vi "Main.vi"(8 "error in (no error)":errorcluster, 10 "Temperature_Notifier":refnum<notifier>, 11 "Message Queues":T1) -> (0 "error out":errorcluster)   [LabVIEW 2019, in "USB-87P8_Manager.lvlib"]
uses:
  USB-87P8_Manager.lvlib
  Framework/Message Queue/All Message Queues.ctl
  Framework/Message Queue/Message Cluster.ctl
  Actor/USB-87Pn_Data.ctl
  USB-87Pn.lvclass
  <vilib>/Utility/sysdir.llb/System Directory Type.ctl
  Framework/Message Queue/Enqueue Message (Single).vi
  Framework/Message Queue/Message Queue.lvlib
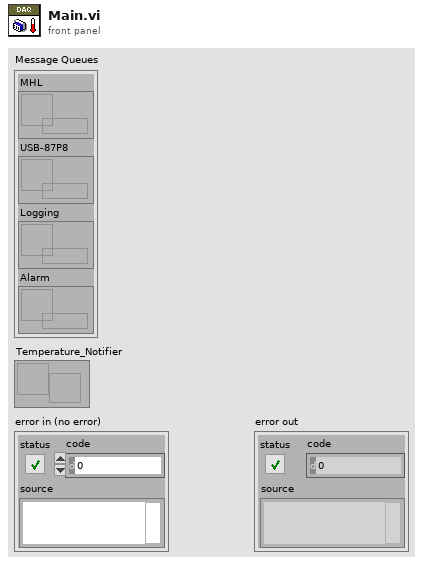
[diagram p1: front panel]
types:
  T1 = typedef "Message Queue.lvlib/All Message Queues.ctl" = cluster{"MHL":refnum<queue>, "USB-87P8":refnum<queue>, "Logging":refnum<queue>, "Alarm":refnum<queue>}
  T2 = typedef "USB-87P8_Manager.lvlib/USB-87Pn_Data.ctl" = cluster{"USB-87Pn":refnum<class "USB-87Pn.lvclass">, "Config_Base_Path":path, "COM Port":i32, "Running?":bool}
  T3 = typedef "System Directory Type.ctl" = i32
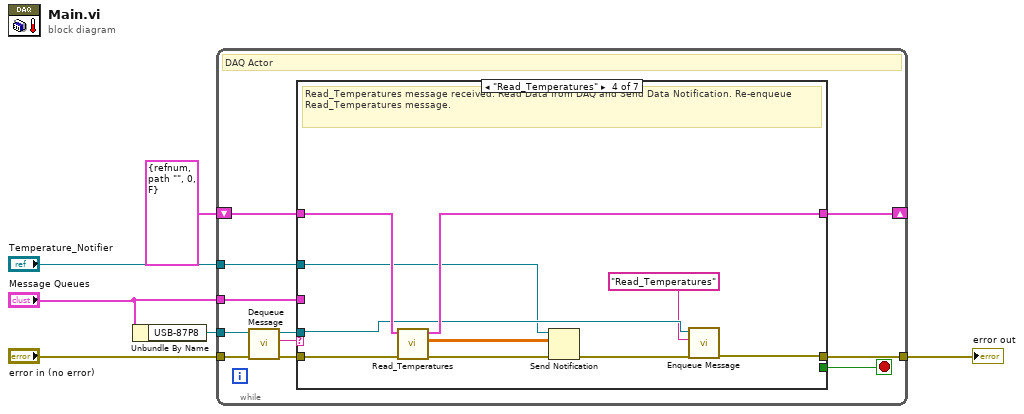
[diagram p0: block diagram]
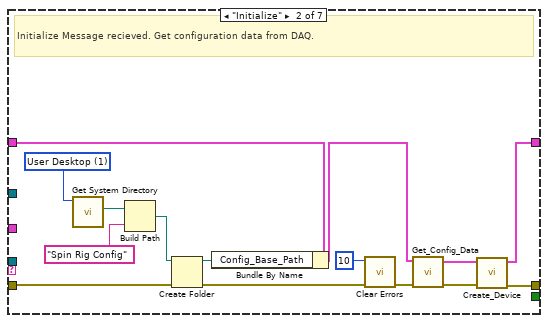
[diagram p3: hidden frame]
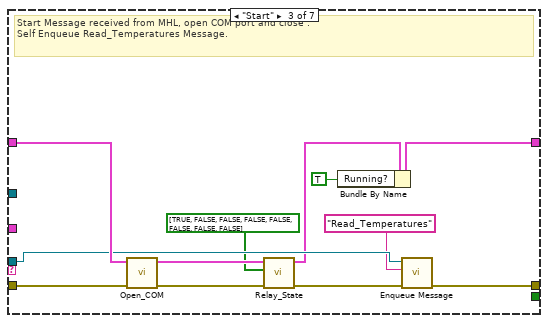
[diagram p4: hidden frame]
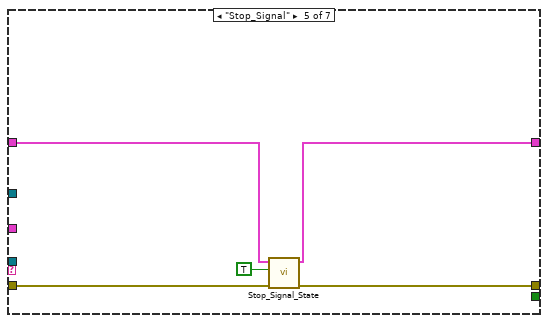
[diagram p5: hidden frame]
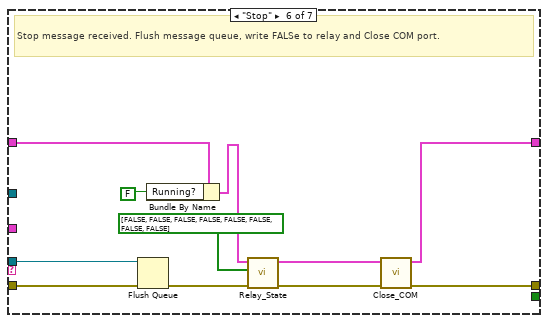
[diagram p6: hidden frame]
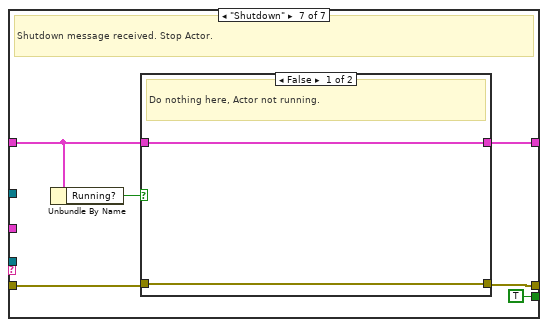
[diagram p7: hidden frame]
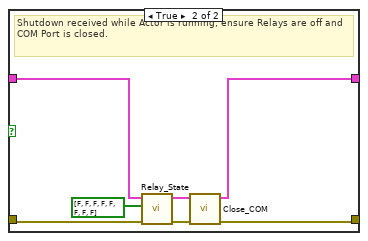
[diagram p8: hidden frame]
diagram:
  n1 = Unbundle By Name("Message Queues") -> ("USB-87P8"=w4:refnum<queue>)
  n2 = while {
    tunnel: "error in (no error)" -> [w17]
    tunnel: "Message Queues" -> [w12]
    tunnel: w4 -> [w16]
    tunnel: [w11] -> w3
    shift-right: [w8] -> _
    shift-left: T2 {"USB-87Pn"=refnum, "Config_Base_Path"=path "", "COM Port"=0, "Running?"=FALSE} -> [w9]
    tunnel: "Temperature_Notifier" -> [w7]
    stop <- w10 stop-if-true
    # "DAQ Actor"
    n3 = call "Dequeue Message.vi"("error in (no error)"=w17, "Message Queue"=w16) -> ("error out"=w13:errorcluster, "Message"=w14:string, "dup Message Queue"=w15:refnum<queue>)  [unwired: 6 in, 1 out]
    n4 = case shown="\"Read_Temperatures\"" w14 {
      tunnel: w15 -> [_ _ w44 w53 _ w72 _]
      tunnel: w13 -> [w19 w24 w45 w55 w58 w71 w77]
      tunnel: w12 -> [_ _ _ _ _ _ _]
      tunnel: [w19 w31 w42 w51 w57 w70 w76] -> w11
      tunnel: [_ _ _ _ _ _ TRUE] -> w10
      tunnel: w9 -> [w18 w22 w46 w56 w61 w64 w74]
      tunnel: [w18 w32 w36 w54 w59 w69 w75] -> w8
      tunnel: w7 -> [_ _ _ w49 _ _ _]
      frame Default {
      }
      frame "Initialize" {
        w28 = T3 1 items=["User Home"=0, "User Desktop"=1, "User Documents"=2, "User Application Data"=3, "User Preferences"=4, "User Temporary"=5, "Public Documents"=6, "Public Application Data"=7, "Public Preferences"=8, "Public Cache"=13, "System Core Libraries"=9, "System Installed Libraries"=10, "Application Files"=11, "Boot Volume Root"=12] ("system directory type")
        # "Initialize Message recieved. Get configuration data from DAQ."
        n5 = call <vilib>:"Get System Directory.vi"("system directory type"=w28) -> ("system directory"=w27:path)  [unwired: 10 in]
        n6 = Build Path(base path=w27, name or relative path="Spin Rig Config") -> (appended path=w26:path)
        n7 = Create Folder(path (use dialog)=w26, error in=w24) -> (created path=w20:path, error out=w23:errorcluster)  [unwired: 1 in, 1 out]
        n8 = Bundle By Name(cluster=w22, "Config_Base_Path"=w20) -> (w21:T2)
        n9 = call <vilib>:"Clear Errors.vi"("error in (no error)"=w23, "specific error code to clear (0: all)"=10) -> ("error out"=w30:errorcluster)  [unwired: 4 in, 1 out]
        n10 = call "Get_Config_Data.vi"("error in (no error)"=w30, "USB-87Pn_Data In"=w21) -> ("error out"=w33:errorcluster, "USB-87Pn_Data Out"=w34:T2)  [unwired: 8 in]
        n11 = call "Create_Device.vi"("error in (no error)"=w33, "USB-87Pn_Data In"=w34) -> ("error out"=w31:errorcluster, "USB-87Pn_Data Out"=w32:T2)  [unwired: 8 in]
      }
      frame "Start" {
        # "Start Message received from MHL, open COM port and close .\nSelf Enqueue Read_Temperatures Message."
        n12 = call "Open_COM.vi"("error in (no error)"=w45, "USB-87Pn_Data In"=w46) -> ("error out"=w41:errorcluster, "USB-87Pn_Data Out"=w39:T2)  [unwired: 8 in]
        n13 = call "Relay_State.vi"("error in (no error)"=w41, "Relay_States"=bool[] [TRUE, FALSE, FALSE, FALSE, FALSE, FALSE, FALSE, FALSE], "USB-87Pn_Data In"=w39) -> ("error out"=w40:errorcluster, "USB-87Pn_Data Out"=w37:T2)  [unwired: 7 in]
        n14 = Bundle By Name(cluster=w37, "Running?"=TRUE) -> (w36:T2)
        n15 = call-poly "Enqueue Message.vi"("error in (no error)"=w40, "Message"="Read_Temperatures", "Message Queue"=w44) -> ("error out"=w42:errorcluster)  [unwired: 7 in, 1 out]
      }
      frame "Read_Temperatures" {
        # "Read_Temperatures message received. Read Data from DAQ and Send Data Notification. Re-enqueue Read_Temperatures message."
        n16 = call "Read_Temperatures.vi"("error in (no error)"=w55, "USB-87Pn_Data In"=w56) -> ("error out"=w50:errorcluster, "Temperature Data"=w48:sgl[][], "USB-87Pn_Data Out"=w54:T2)  [unwired: 7 in]
        n17 = Send Notification(notification=w48, notifier=w49, error in (no error)=w50) -> (error out=w47:errorcluster)  [unwired: 1 out]
        n18 = call-poly "Enqueue Message.vi"("error in (no error)"=w47, "Message"="Read_Temperatures", "Message Queue"=w53) -> ("error out"=w51:errorcluster)  [unwired: 7 in, 1 out]
      }
      frame "Stop_Signal" {
        n19 = call "Stop_Signal_State.vi"("error in (no error)"=w58, "Stop Signal"=TRUE, "USB-87Pn_Data"=w61) -> ("error out"=w57:errorcluster, "USB-87Pn_Data out"=w59:T2)  [unwired: 7 in]
      }
      frame "Stop" {
        # "Stop message received. Flush message queue, write FALSe to relay and Close COM port."
        n20 = Flush Queue(queue=w72, error in (no error)=w71) -> (error out=w67:errorcluster)  [unwired: 2 out]
        n21 = Bundle By Name(cluster=w64, "Running?"=FALSE) -> (w63:T2)
        n22 = call "Relay_State.vi"("error in (no error)"=w67, "Relay_States"=bool[] [FALSE, FALSE, FALSE, FALSE, FALSE, FALSE, FALSE, FALSE], "USB-87Pn_Data In"=w63) -> ("error out"=w66:errorcluster, "USB-87Pn_Data Out"=w68:T2)  [unwired: 7 in]
        n23 = call "Close_COM.vi"("error in (no error)"=w66, "USB-87Pn_Data In"=w68) -> ("error out"=w70:errorcluster, "USB-87Pn_Data out"=w69:T2)  [unwired: 8 in]
      }
      frame "Shutdown" {
        # "Shutdown message received. Stop Actor."
        n24 = Unbundle By Name(w74) -> ("Running?"=w73:bool)
        n25 = case shown="False" w73 {
          tunnel: w77 -> [w79 w85]
          tunnel: [w79 w84] -> w76
          tunnel: [w80 w82] -> w75
          tunnel: w74 -> [w80 w81]
          frame False {
            # "Do nothing here, Actor not running."
          }
          frame True {
            # "Shutdown received while Actor is running, ensure Relays are off and COM Port is closed."
            n26 = call "Relay_State.vi"("error in (no error)"=w85, "Relay_States"=bool[] [FALSE, FALSE, FALSE, FALSE, FALSE, FALSE, FALSE, FALSE], "USB-87Pn_Data In"=w81) -> ("error out"=w83:errorcluster, "USB-87Pn_Data Out"=w87:T2)  [unwired: 7 in]
            n27 = call "Close_COM.vi"("error in (no error)"=w83, "USB-87Pn_Data In"=w87) -> ("error out"=w84:errorcluster, "USB-87Pn_Data out"=w82:T2)  [unwired: 8 in]
          }
        }
      }
    }
  }
  "error out" <- w3
